vi "Moving Average_AB.vi"(9 "Filter Width":i32, 11 "Input Array":dbl[][](array[numeric])) -> (3 "Moving Averaged Array":dbl[][](array[numeric]))   [LabVIEW 2018]
uses:
  <vilib>/ptbypt/NI_PtbyPt.lvlib
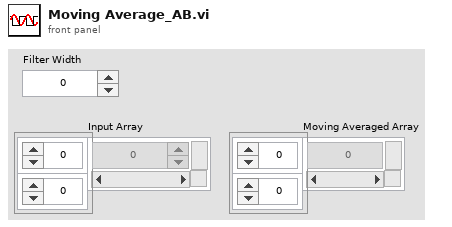
[diagram p1: front panel]
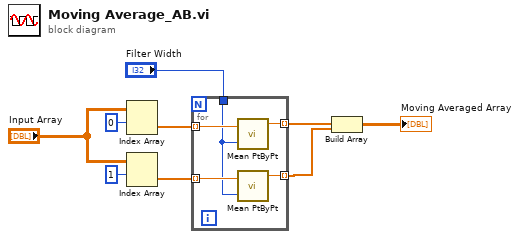
[diagram p0: block diagram]
diagram:
  n1 = Index Array(array="Input Array", index (row)=0) -> (element=w7:dbl[])  [unwired: 1 in]
  n2 = Index Array(array="Input Array", index (row)=1) -> (element=w6:dbl[])  [unwired: 1 in]
  n3 = for {
    tunnel: w7 -> [w14] mode=indexing
    tunnel: w6 -> [w13] mode=indexing
    tunnel: [w12] -> w4 mode=indexing
    tunnel: [w11] -> w3 mode=indexing
    tunnel: "Filter Width" -> [w10]
    n4 = call <vilib>:"Mean PtByPt.vi"("x"=w14, "sample length"=w10) -> ("mean"=w12:dbl)  [unwired: 2 in, 1 out]
    n5 = call <vilib>:"Mean PtByPt.vi"("x"=w13, "sample length"=w10) -> ("mean"=w11:dbl)  [unwired: 2 in, 1 out]
  }
  n6 = Build Array(w4, w3) -> (→"Moving Averaged Array":dbl[][])
